vi "Login.vi"(8 "error in":errorcluster, 10 "Login":bool, 11 "Base Software in":refnum<class "Main.lvclass">) -> (0 "error out":errorcluster, 3 "Base Software out":refnum<class "Main.lvclass">)   [LabVIEW 2023, in "Main.lvlib" / "Main.lvclass"]
uses:
  Project/Main.lvclass
  Project/Main.lvclass/Main.ctl
  builds/Engine/Engine.lvlibp/Project/Engine.lvclass
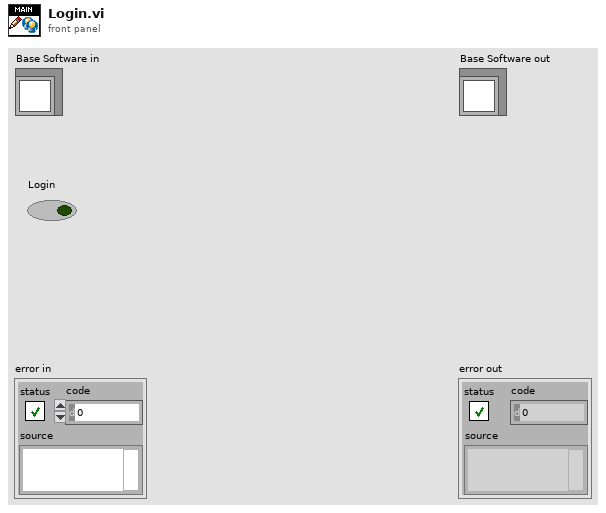
[diagram p1: front panel]
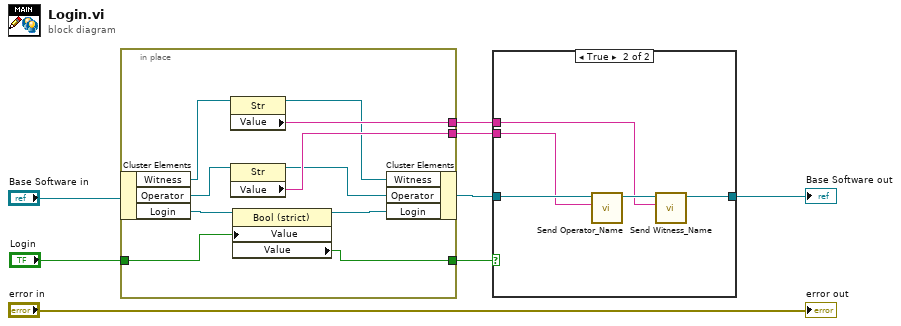
[diagram p0: block diagram]
diagram:
  n1 = in-place {
    in-place-border: "Login" -> [w18]
    in-place-border: [w11] -> w5
    in-place-border: [w17] -> w2
    in-place-border: [w16] -> w1
    n2 = in-place-cluster #1("Base Software in") -> ("Witness"=w15:refnum<vi>, "Operator"=w14:refnum<vi>, "Login"=w13:refnum<vi>)
    n3 = property class="Str"(reference=w15) -> (reference out=w9:refnum<vi>, "Value"=w17:string)  [unwired: 1 in, 1 out]
    n4 = property class="Str"(reference=w14) -> (reference out=w10:refnum<vi>, "Value"=w16:string)  [unwired: 1 in, 1 out]
    n5 = property class="Bool (strict)"(reference=w13, "Value"=w18) -> (reference out=w12:refnum<vi>, "Value"=w11:bool)  [unwired: 1 in, 1 out]
    n6 = in-place-cluster #1("Witness"=w9, "Operator"=w10, "Login"=w12) -> (w4:refnum<class "Main.lvclass">)
  }
  n7 = case shown="True" w5 {
    tunnel: w4 -> [w19 w22]
    tunnel: [w19 w23] -> w3
    tunnel: w2 -> [_ w21]
    tunnel: w1 -> [_ w20]
    frame False {
    }
    frame True {
      n8 = call "Send Operator_Name.vi"("Operator Name"=w20, "Engine in"=w22) -> ("Engine out"=w24:refnum<class "Main.lvclass">)  [unwired: 8 in, 1 out]
      n9 = call "Send Witness_Name.vi"("Witness Name"=w21, "Engine in"=w24) -> ("Engine out"=w23:refnum<class "Main.lvclass">)  [unwired: 8 in, 1 out]
    }
  }
  "Base Software out" <- w3
  "error out" <- "error in"
